vi "decompress_incoming_data_Rev01.vi"(8 "N":dbl, 9 "Input Data":u8[](array[numeric])=[63, 21]) -> (3 "Combined output binary values":u8[](array[numeric]) format="%08b")   [LabVIEW 2012]
panel:
  out "Packed byte":u8[](array[numeric]) format="%08b"
  out "LSB Array size":i32
  out "MSB Array size":i32
  out "array 0 size":dbl
  out "3Byte array":u8[](array[numeric])
  out "Byte 2 array":u8[](array[numeric])
  out "Byte 1 array":u8[](array[numeric])
  out "Byte 0 array":u8[](array[numeric])
  out "Input Array Size":dbl
  out "Loop count":i32
  out "Byte 2":bool[](array[boolean])
  out "Byte 1":bool[](array[boolean])
  out "Byte 0":bool[](array[boolean])
  out "The last input byte":bool[](array[boolean])
  out "Loop Counter":dbl
  # "Each incoming byte from 0 - 2047 has 3 bytes of data"
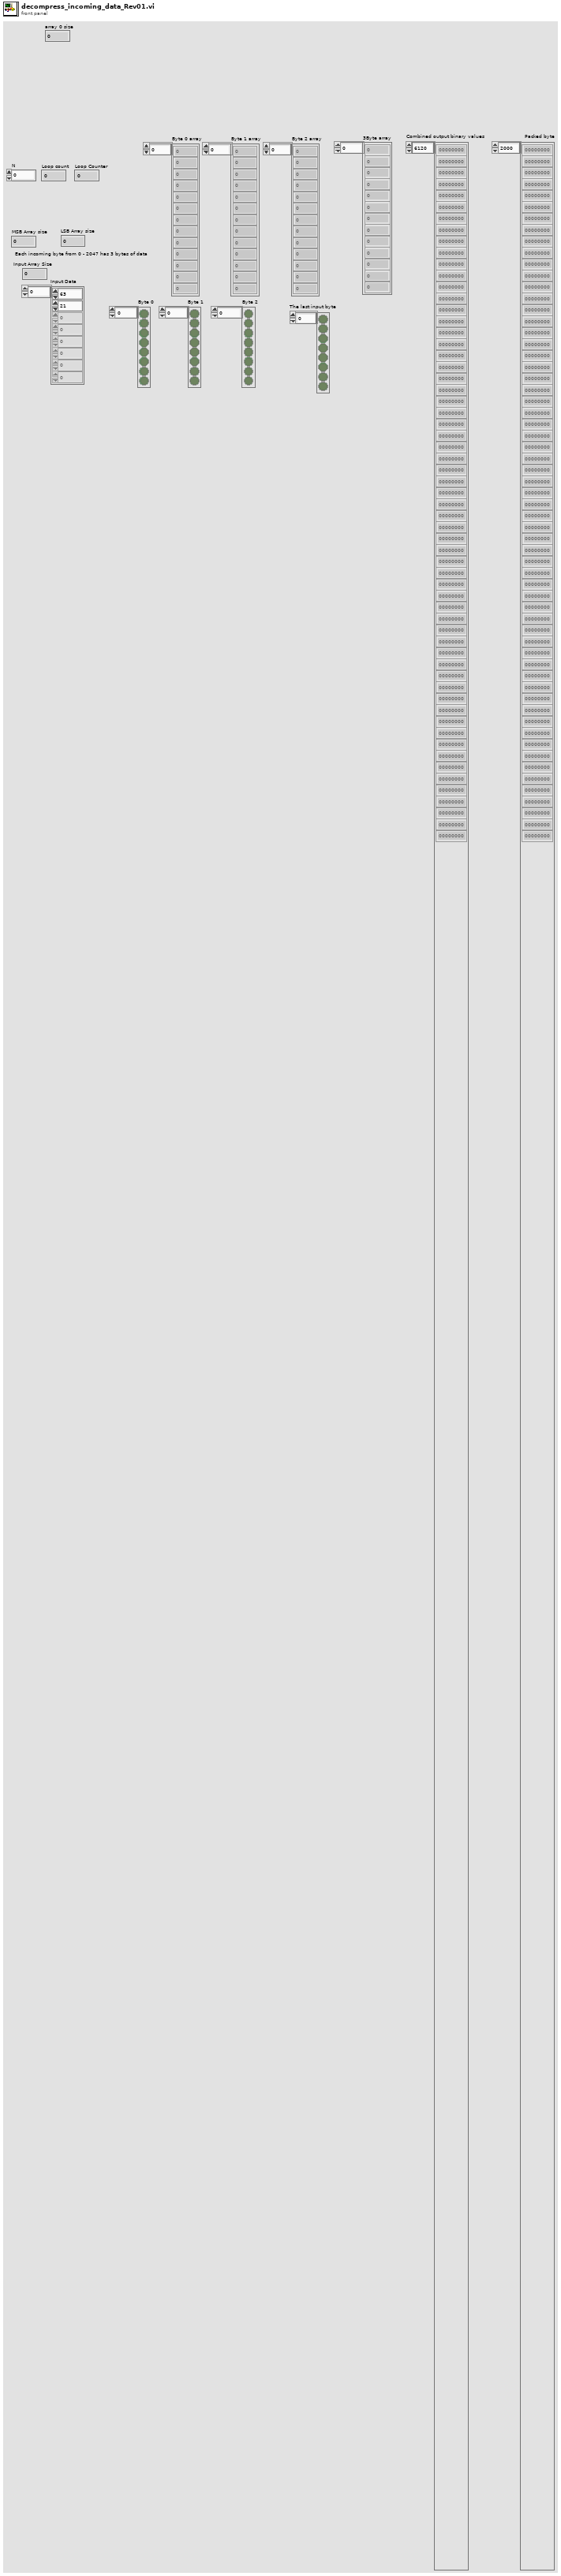
[diagram p1: front panel]
types:
  T1 = cluster{"Boolean array[0]":bool, "Boolean array[1]":bool, "Boolean array[2]":bool, "Boolean array[3]":bool, "Boolean array[4]":bool, "Boolean array[5]":bool, "Boolean array[6]":bool, "Boolean array[7]":bool}
  T2 = cluster{"Boolean array[0]":bool, "Boolean array[1]":bool, bool, bool, bool, bool, bool, bool}
  T3 = cluster{"Boolean array[2]":bool, "Boolean array[3]":bool, bool, bool, bool, bool, bool, bool}
  T4 = cluster{"Boolean array[4]":bool, "Boolean array[5]":bool, bool, bool, bool, bool, bool, bool}
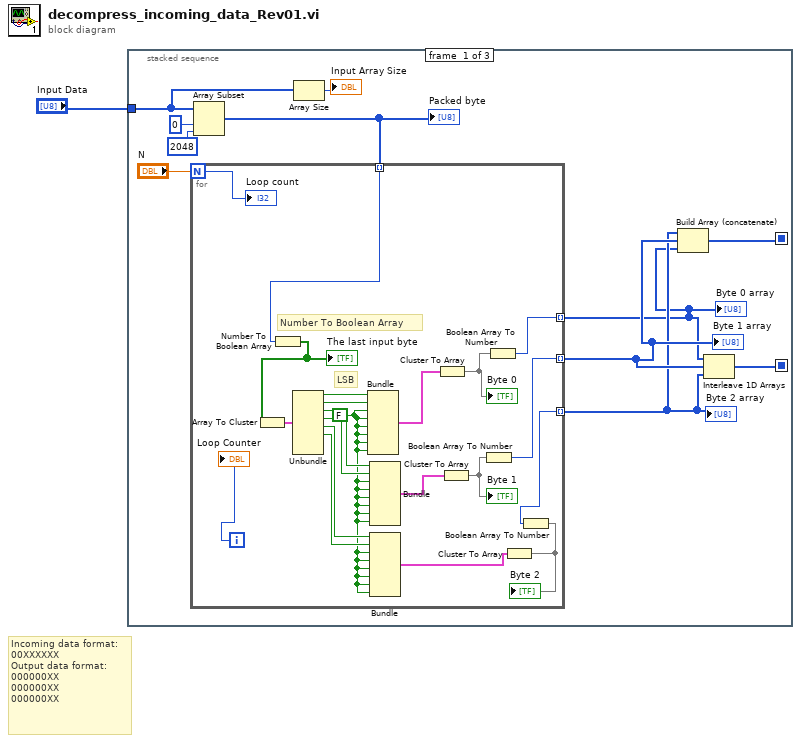
[diagram p0: block diagram]
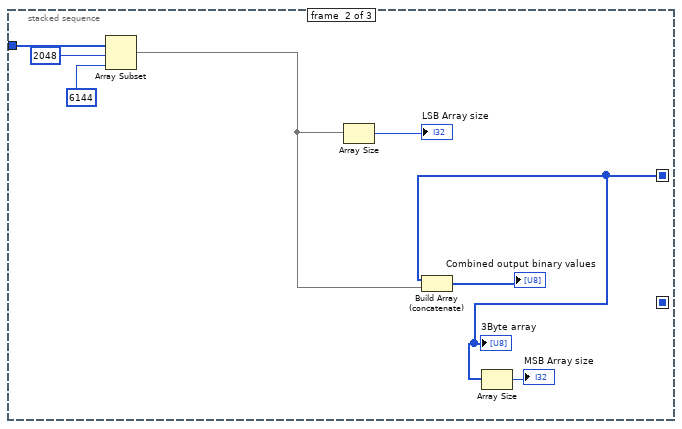
[diagram p2: hidden frame]
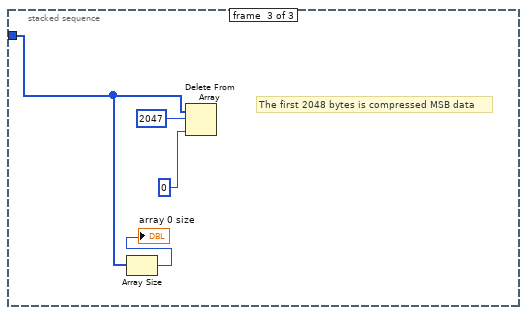
[diagram p3: hidden frame]
diagram:
  # "Incoming data format:\n00XXXXXX\nOutput data format:\n000000XX\n000000XX\n000000XX"
  n1 = stacked-sequence {
    seq-local: [w10 _ _] -> [_ _ _]
    seq-local: [w4 _ _] -> [_ w34 _]
    tunnel: "Input Data" -> [w7 w38 w42]
    frame #0 {
      n2 = Array Subset(array=w7, index=0, length=2048) -> (w6:u8[])
      "Packed byte" <- w6
      n3 = for {
        N: "N" -> [w23]
        tunnel: [w13] -> w3 mode=indexing
        tunnel: w6 -> [w16] mode=indexing
        tunnel: [w15] -> w2 mode=indexing
        tunnel: [w14] -> w5 mode=indexing
        i -> [w19]
        w20 = FALSE
        # "Number To Boolean Array"
        # "LSB"
        n4 = Number To Boolean Array(number=w16) -> (Boolean array=w26:bool[])
        "The last input byte" <- w26
        n5 = Array To Cluster(array=w26) -> (cluster=w27:T1)
        n6 = Unbundle(w27) -> ("Boolean array[0]"=w33:bool, "Boolean array[1]"=w32:bool, "Boolean array[2]"=w31:bool, "Boolean array[3]"=w30:bool, "Boolean array[4]"=w29:bool, "Boolean array[5]"=w28:bool)  [unwired: 2 out]
        n7 = Bundle("Boolean array[0]"=w33, "Boolean array[1]"=w32, w20, w20, w20, w20, w20, w20) -> (w17:T2)  [unwired: 1 in]
        n8 = Bundle("Boolean array[2]"=w31, "Boolean array[3]"=w30, w20, w20, w20, w20, w20, w20) -> (w22:T3)  [unwired: 1 in]
        n9 = Bundle("Boolean array[4]"=w29, "Boolean array[5]"=w28, w20, w20, w20, w20, w20, w20) -> (w21:T4)  [unwired: 1 in]
        n10 = Cluster To Array(cluster=w17) -> (array=w18:bool[])
        "Byte 0" <- w18
        n11 = Cluster To Array(cluster=w22) -> (array=w25:bool[])
        "Byte 1" <- w25
        n12 = Boolean Array To Number(Boolean array=w25) -> (number=w14:u8)
        n13 = Boolean Array To Number(Boolean array=w18) -> (number=w15:u8)
        n14 = Cluster To Array(cluster=w21) -> (array=w24:bool[])
        "Byte 2" <- w24
        n15 = Boolean Array To Number(Boolean array=w24) -> (number=w13:u8)
        "Loop Counter" <- w19
        "Loop count" <- w23
      }
      "Byte 0 array" <- w2
      "Byte 1 array" <- w5
      "Byte 2 array" <- w3
      n16 = Array Size(array=w7) -> (size(s)=→"Input Array Size":i32)
      n17 = Build Array (concatenate)(w3, w5, w2) -> (w4:u8[])
      n18 = Interleave 1D Arrays(w2, w5, w3) -> (w10:u8[])
    }
    frame #1 {
      n19 = Array Subset(array=w38, index=2048, length=6144) -> (w35:u8[])
      n20 = Array Size(array=w35) -> (size(s)=→"LSB Array size":i32)
      n21 = Build Array (concatenate)(w34, w35) -> (→"Combined output binary values":u8[])
      n22 = Array Size(array=w34) -> (size(s)=→"MSB Array size":i32)
      "3Byte array" <- w34
    }
    frame #2 {
      # "The first 2048 bytes is compressed MSB data"
      n23 = Array Size(array=w42) -> (size(s)=→"array 0 size":i32)
      n24 = Delete From Array(array=w42, length=2047, index=0) -> ()  [unwired: 2 out]
    }
  }
